vi "Stop Streaming.vi"(8 "error in (no error)":errorcluster, 11 "Synchronization Device in":refnum<class "Arduino DAQ.lvclass">) -> (0 "error out":errorcluster, 3 "Synchronization Device out":refnum<class "Arduino DAQ.lvclass">)   [LabVIEW 2023, in "Arduino DAQ.lvlib" / "Arduino DAQ.lvclass"]
uses:
  Arduino DAQ.lvclass
  Arduino DAQ.lvclass/Arduino DAQ.ctl
  Arduino DAQ.lvlib
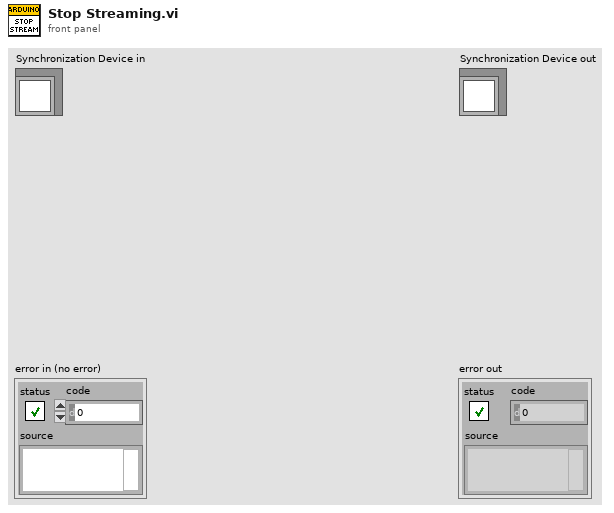
[diagram p1: front panel]
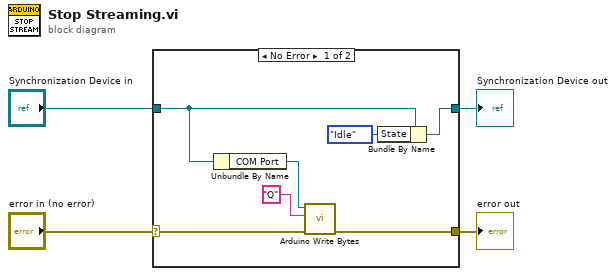
[diagram p0: block diagram]
diagram:
  n1 = case shown="No Error" "error in (no error)" {
    selector: "error in (no error)" -> [w11 w13]
    tunnel: [w8 w13] -> w3
    tunnel: [w5 w12] -> w1
    tunnel: "Synchronization Device in" -> [w6 w12]
    frame No Error {
      n2 = Unbundle By Name(w6) -> ("COM Port"=w10:refnum<visa-resource-name>)
      n3 = call "Arduino Write Bytes.vi"("error in (no error)"=w11, "Command"="Q", "COM Port In"=w10) -> ("error out"=w8:errorcluster)  [unwired: 7 in, 1 out]
      n4 = Bundle By Name(cluster=w6, "State"=enum16{"Idle", "Manual", "Stream"}."Idle") -> (w5:refnum<class "Arduino DAQ.lvclass">)
    }
    frame Error {
    }
  }
  "error out" <- w3
  "Synchronization Device out" <- w1
